vi "Combine_3Ghz.vi"(8 "Over? Array AI0":bool[](array[boolean])=[FALSE, FALSE, FALSE, FALSE, FALSE, FALSE, FALSE, FALSE], 9 "Over? Array AI1":bool[](array[boolean])=[FALSE, FALSE, FALSE, FALSE, FALSE, FALSE, FALSE, FALSE], 10 "A0 cluster in":T2, 11 "A1 cluster in":T2) -> (0 "Over? Array Out":bool[](array[boolean]), 3 "A0 cluster out":T1)   [LabVIEW 2014]
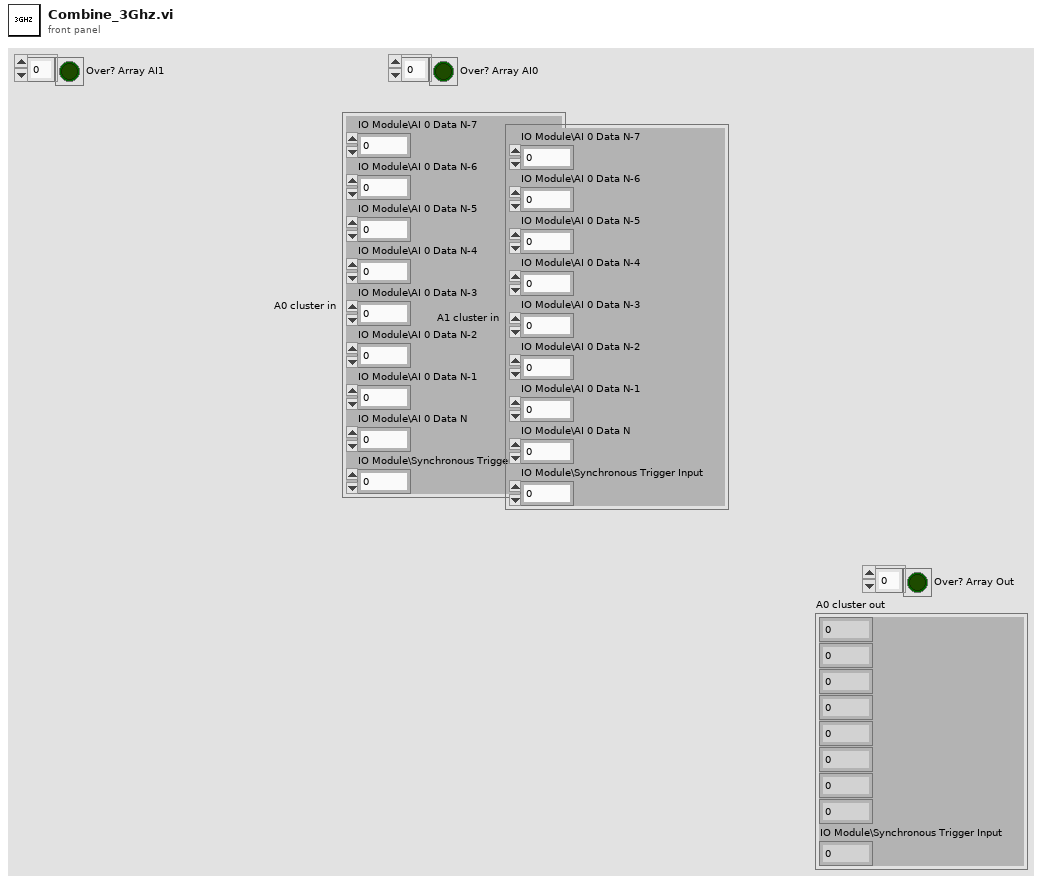
[diagram p1: front panel]
types:
  T1 = cluster{u16, u16, u16, u16, u16, u16, u16, u16, "IO Module\\Synchronous Trigger Input":u8}
  T2 = cluster{"IO Module\\AI 0 Data N-7":u8, "IO Module\\AI 0 Data N-6":u8, "IO Module\\AI 0 Data N-5":u8, "IO Module\\AI 0 Data N-4":u8, "IO Module\\AI 0 Data N-3":u8, "IO Module\\AI 0 Data N-2":u8, "IO Module\\AI 0 Data N-1":u8, "IO Module\\AI 0 Data N":u8, "IO Module\\Synchronous Trigger Input":u8}
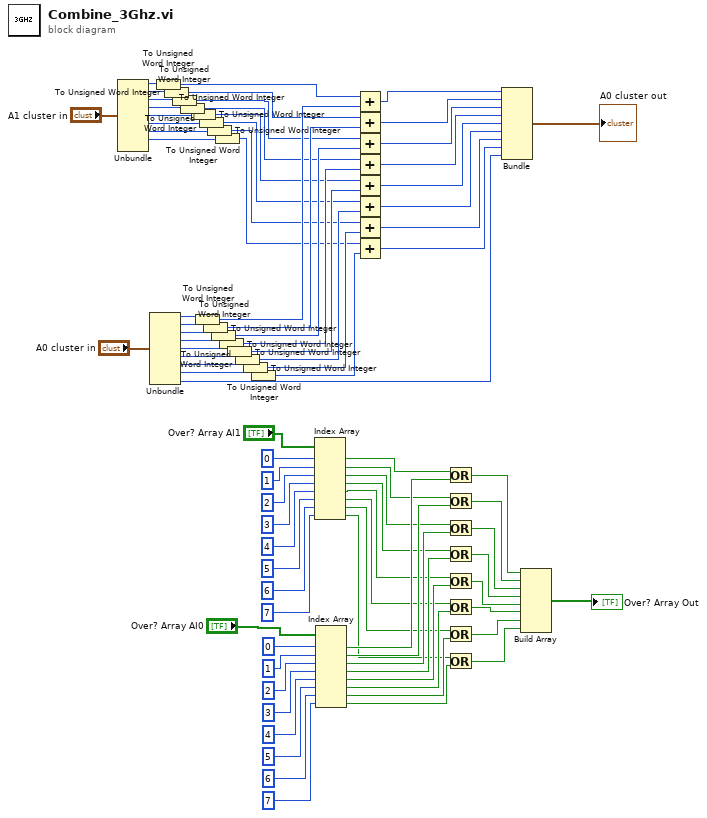
[diagram p0: block diagram]
diagram:
  n1 = Unbundle("A1 cluster in") -> ("IO Module\\AI 0 Data N-7"=w3:u8, "IO Module\\AI 0 Data N-6"=w5:u8, "IO Module\\AI 0 Data N-5"=w7:u8, "IO Module\\AI 0 Data N-4"=w9:u8, "IO Module\\AI 0 Data N-3"=w11:u8, "IO Module\\AI 0 Data N-2"=w13:u8, "IO Module\\AI 0 Data N-1"=w15:u8, "IO Module\\AI 0 Data N"=w17:u8)  [unwired: 1 out]
  n2 = Unbundle("A0 cluster in") -> ("IO Module\\AI 0 Data N-7"=w19:u8, "IO Module\\AI 0 Data N-6"=w21:u8, "IO Module\\AI 0 Data N-5"=w23:u8, "IO Module\\AI 0 Data N-4"=w25:u8, "IO Module\\AI 0 Data N-3"=w27:u8, "IO Module\\AI 0 Data N-2"=w29:u8, "IO Module\\AI 0 Data N-1"=w31:u8, "IO Module\\AI 0 Data N"=w33:u8, "IO Module\\Synchronous Trigger Input"=w34:u8)
  n3 = To Unsigned Word Integer(number=w3) -> (unsigned 16bit integer=w2:u16)
  n4 = To Unsigned Word Integer(number=w5) -> (unsigned 16bit integer=w4:u16)
  n5 = To Unsigned Word Integer(number=w7) -> (unsigned 16bit integer=w6:u16)
  n6 = To Unsigned Word Integer(number=w9) -> (unsigned 16bit integer=w8:u16)
  n7 = To Unsigned Word Integer(number=w11) -> (unsigned 16bit integer=w10:u16)
  n8 = To Unsigned Word Integer(number=w19) -> (unsigned 16bit integer=w18:u16)
  n9 = To Unsigned Word Integer(number=w13) -> (unsigned 16bit integer=w12:u16)
  n10 = To Unsigned Word Integer(number=w21) -> (unsigned 16bit integer=w20:u16)
  n11 = To Unsigned Word Integer(number=w15) -> (unsigned 16bit integer=w14:u16)
  n12 = To Unsigned Word Integer(number=w23) -> (unsigned 16bit integer=w22:u16)
  n13 = To Unsigned Word Integer(number=w17) -> (unsigned 16bit integer=w16:u16)
  n14 = To Unsigned Word Integer(number=w25) -> (unsigned 16bit integer=w24:u16)
  n15 = To Unsigned Word Integer(number=w27) -> (unsigned 16bit integer=w26:u16)
  n16 = To Unsigned Word Integer(number=w29) -> (unsigned 16bit integer=w28:u16)
  n17 = To Unsigned Word Integer(number=w31) -> (unsigned 16bit integer=w30:u16)
  n18 = To Unsigned Word Integer(number=w33) -> (unsigned 16bit integer=w32:u16)
  n19 = Index Array(array="Over? Array AI1", index #1=0 ("index"), index #2=1 ("index"), index #3=2 ("index"), index #4=3 ("index"), index #5=4 ("index"), index #6=5 ("index"), index #7=6 ("index"), index #8=7 ("index")) -> (element #1=w67:bool, element #2=w65:bool, element #3=w63:bool, element #4=w61:bool, element #5=w59:bool, element #6=w57:bool, element #7=w55:bool, element #8=w52:bool)
  n20 = Index Array(array="Over? Array AI0", index #1=0 ("index"), index #2=1 ("index"), index #3=2 ("index"), index #4=3 ("index"), index #5=4 ("index"), index #6=5 ("index"), index #7=6 ("index"), index #8=7 ("index")) -> (element #1=w66:bool, element #2=w64:bool, element #3=w62:bool, element #4=w60:bool, element #5=w58:bool, element #6=w56:bool, element #7=w54:bool, element #8=w53:bool)
  n21 = Add(x=w2, y=w18) -> (x+y=w42:u16)
  n22 = Add(x=w4, y=w20) -> (x+y=w41:u16)
  n23 = Add(x=w6, y=w22) -> (x+y=w40:u16)
  n24 = Add(x=w8, y=w24) -> (x+y=w39:u16)
  n25 = Add(x=w10, y=w26) -> (x+y=w38:u16)
  n26 = Add(x=w12, y=w28) -> (x+y=w37:u16)
  n27 = Add(x=w14, y=w30) -> (x+y=w36:u16)
  n28 = Add(x=w16, y=w32) -> (x+y=w35:u16)
  n29 = Or(x=w67, y=w66) -> (x .or. y?=w51:bool)
  n30 = Or(x=w65, y=w64) -> (x .or. y?=w50:bool)
  n31 = Or(x=w63, y=w62) -> (x .or. y?=w49:bool)
  n32 = Or(x=w61, y=w60) -> (x .or. y?=w48:bool)
  n33 = Or(x=w59, y=w58) -> (x .or. y?=w47:bool)
  n34 = Or(x=w57, y=w56) -> (x .or. y?=w46:bool)
  n35 = Or(x=w55, y=w54) -> (x .or. y?=w45:bool)
  n36 = Or(x=w52, y=w53) -> (x .or. y?=w44:bool)
  n37 = Bundle(w42, w41, w40, w39, w38, w37, w36, w35, "IO Module\\Synchronous Trigger Input"=w34) -> (→"A0 cluster out":T1)  [unwired: 1 in]
  n38 = Build Array(w51, w50, w49, w48, w47, w46, w45, w44) -> (→"Over? Array Out":bool[])
